vi "2023_day16_Task1.vi"() -> ()   [LabVIEW 2021]
uses:
  45de9bef-49e1-442e-b527-3241b48d18bf.vi
panel:
  out "Task 1":i32
  in  "Switch":bool caption="Ex. Data  vs.  User Data"
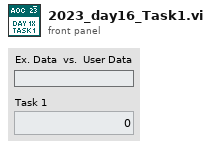
[diagram p1: front panel]
types:
  T1 = cluster{"Map":string[][], "Direction":enum16{"UP", "LEFT", "DOWN", "RIGHT"}, "Position (Row,Col)":i32[], "Energized Tiles":i32[][]}
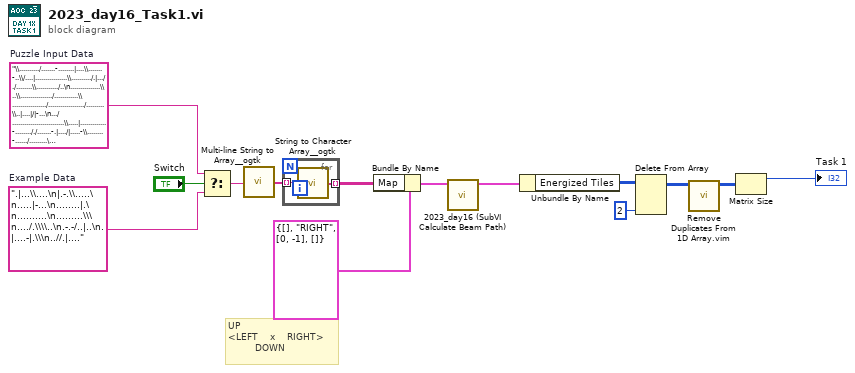
[diagram p0: block diagram]
diagram:
  w12 = "\\........../.......-........|....\\.......-..\\/....|................\\........../.|..././........\\.........../..\n...............\\..\\................/............\\................./................../.........\\..|....|/|-...\n.../..........................\\.....|.............-.......././.......-.|..../|.....-\\........-....../.........\n|..........................-..........-......./............................-..|................-..............\n.....|......../...../.......-.\\..............................-........|............|/.../../........./........\n..\\...|..-......\\.........-\\.||........|./................\\....\\........-..\\..................../..\\....-...|.\n.|...........|............-........./.-.................|.|....../...............|..../..-..-...\\...........|.\n..............\\............................................................./......................./\\....-...\n./........|...\\.\\..|..-....\\............................|........./.................|/...............-........\n\\....\\./.............../................../....|......./........../.\\......./........-....\\......../....../|..\n./......--..........\\..|.--........-...../......./........\\.....|/..................|//...........|.........-.\n.......|.....\\-.\\..-......-.........|.....................-/\\.....-..........|.............-....\\.....\\.-.....\n..--...\\....-..|..................................-......-......\\......-................\\...../..-/....--.....\n....-.........................\\.\\............|...............|.....-...\\....|-................................\n.................-..|.\\..\\....-..........|...../.....-...-.-../.............../................-..............\n-..-......|..............................\\.....\\........|...../........\\.................../..................\n..............-.....-.|..........|.\\..................|........|...........\\.\\...|........-...................\n..\\............/...\\\\........../...-..\\.../.........\\..|................../......\\..-.../....................\\\n..................|...\\......................./...|......../..............-./...\\........\\......./|...\\..-..-.\n.................................................-................|.........................................\\.\n......-...............................|./............./...........................-\\/..../......\\..........\\..\n......\\....|..........................\\.-|..........................|....................\\.....\\/...-.........\n..\\..-|...|.....-...../......./....|...............\\................|..|.......\\...........................-..\n..\\......-.......\\.........\\................|...........|....../...../..........-./...-|..................../.\n................./.......\\...|.....\\....-................./......../..\\...........-...|.../|................\\.\n..|..\\./.........\\.\\.......................-......|....-..../.../................-.......\\../.../...../.......\n........../........./..|..-....................\\\\............\\........................-......-......|.........\n.../-....\\..\\..........\\....\\\\......................................./........\\...-.................\\.........\n................................../.................|..\\.-..|................|/....-.........................|\n...-.................||..../....................-..........................................|.-................\n..//.\\..........................|.....|-.............\\.\\......-....\\.\\.......\\............-..............\\-...\n.......|.|..-........./..|........-.....|........................-...................-......\\................-\n..-..|..........|....-.............|.|/...../../..................\\...\\................../......|....|........\n........\\..././.............../.............../....-../.....|....\\................|/.../.....|.|-..|..........\n......|..........\\...-./........-...............................\\..........|.............|..\\..|......./.....|\n.............................-................................................|................/......\\.../..-\n......-........\\..........-..../...............\\............/.....\\......|........................-.|.../.....\n...\\...............-....-........-............-...../....|.\\.../.......\\..-....................|........|.....\n.............................-...\\....|...|.......\\............................-............\\.................\n....................|...-........-.........-..\\................/....................../.|.......-.............\n......\\.........................../....-....|...........................................\\...-.........|......\\\n.............\\../\\..............|\\.\\..........|\\.../..................../\\...................|\\.......\\.......\n/.................../.\\\\.........................../...........-...-..........-..-............................\n............\\......../........-.........../........./.................-................./...........|.........\n.........\\.......|.......\\........./.....................\\..............\\\\....../...|-....\\..|..-.....|.......\n.|....-.............\\.........\\.\\../.......-...........................\\./..........................--\\......\\\n........./..../................./.................\\............................................./../.\\........\n.....-..............-.-...\\/..|....-........./.....................\\................./.\\..........-...|....|..\n........|...|.-.......|.......-............\\.../....|...\\............../............-.........................\n........................|.....\\........................./\\/.........................|.........................\n....\\..././..........|.....\\......................-................./.....|...............................|-..\n.../.........../.-......\\..../.................-...\\.....-......\\.....\\..............//.|..............-..-...\n....../............./-/.\\...........\\...\\..|/........................-...../......\\........-./\\..........||...\n.................................../............|....................../..|.....\\......\\............/.........\n.....|....\\...|.-./............................./..-....|.\\.......................-../.-..-.........\\.........\n..........\\...|../.......-|............-........../...../..........-......-../.-......|..../.-.../............\n.-.........-............|/.......-........|...................-.........-........../.-........\\..........|/...\n.........\\.........\\....../....|...\\\\......-..........-................\\................................-.....\n............-...../......|...//........\\-....|......../........./..................-................../....--.\n...............|.................................|.../...\\....................\\................|...\\.|........\n..............\\.........\\.........\\....|.-.......\\.\\........-.........../...|.....|..............\\.......\\....\n........-.-.....|.../......-\\..|.....-.........|.-................\\......./....\\...-.....\\..|/...............|\n....|.....................-...................\\......\\......-.......................-...../........./....\\....\n..|...|.......\\./..-..............\\.............................................\\../....|.....................\n..................-../........|.....-\\.../................................................./..\\...|......-...-\n.....\\......\\........\\.....................|...|../......../....../.\\........./...............................\n............../........../...........\\..\\/..|.\\...|..........-................................\\-..............\n/...............\\...|......\\............/|...................|....././...\\............................-.|.....\n...........|................/-......\\.....-.........-.............../......./............../|.................\n..-...........|..\\.............\\....|/...............|..../..............\\...............|./......|........./.\n.....\\\\..|......\\....\\.......-.................\\.-......................|........./...|.........|...|...-.....\n-...../....|....../............./.......|/../\\.............../...../-\\.../-.......|........../..............\\\\\n..........\\....................../.................|...--../..................................................\n.\\.................../......|......-.............................//......|.../|.|....\\.............\\..........\n.\\-...........-.........|..................................../........|......../...-............\\....-...-....\n......\\......|................-...../....|........-..\\.....-........//................../.....|.........-.....\n.....-..........-.|/.........-....................../......|.|./........................................./\\\\|.\n...\\................|.........../..-....|..-..........|........../....-....../......./.....-..\\.....\\\\..../...\n.....\\.....-..................-...-..../....|....|.................|...\\./.............../.......|.\\/...../...\n.||......../........../.-...|...........\\.................\\........-........|........................-...|....\n........./......\\......|...............\\.\\.................................................\\.................|\n..........................|....................|..../-...............|....|......../....-..................|..\n.-........\\.|......../...|...................|.........|............\\.....|.......\\........./.................\n................-........................\\...........|................../................-.............\\......\n.......\\..........|.............../...|.-......................../....\\.............-.......\\./...............\n..........\\...........................................-........|.......\\........./...-........\\...............\n../......./...\\|...............-........\\................./...\\...................../.....-.-....-...........-\n.\\../......../....-\\................................|.....-..|...............................-................\n..........................\\.....|................/.....\\......../.............|..............\\......./-..|....\n|.........-.|............./......-.................|.......|...\\/...........|...........................\\\\....\n-..................|.........................-.............-.....|..../.........\\...-/.....|............/\\....\n.........\\.\\....\\...........|....-.../..............|.....|-.......\\.............-......./......././.......\\..\n..../.....-...........................................\\.../..\\.|.......................-..//....-......|......\n./-..................\\..\\....................................\\......./.\\....|.................................\n...../....................................-....-/........................-/.........-.\\...|......./..-.\\......\n.....|.............-.......|-..-.................................|-...........................\\.|.....|.......\n.........\\-.............\\.............../....-....|....-.|..........\\............|.\\...|.....-................\n............/.......-....|./....|../..../......./..\\.................-..................|.....................\n../....-........./.....\\...............\\......-....|...\\........../.....|........................\\............\n...../.\\.............\\.........................-..|.......|......-......|................./......./-..........\n...\\..........\\.......................\\.-..././.........|..\\..................\\...../...|.......|............-\n........./............-..................................|.....................-..............................\n........................|.....\\.........\\..............-..\\..........||...../.\\\\./....../.....................\n.................-.............\\.../...........\\...\\......--................\\.....\\.............\\....-........\n.../-..........\\.\\............-.......-.............\\..\\.\\...../........|...-..-..|..........\\................\n\\.|..\\......\\-......./.........||..\\.........................................................-...../..........\n....|..........................................\\......-..........\\.../...\\-........|..........................\n.......-.......\\..//./....|...............\\.\\..-...\\....|....................-......\\......\\..-......../......\n/..../../....-../....-....-......................\\........./..........-/..\\......./..\\-.../..........|........\n.|....\\\\........./....\\.............-......--\\...........|.........|..\\...................../........./.\\....."  # Puzzle Input Data
  w13 = ".|...\\....\n|.-.\\.....\n.....|-...\n........|.\n..........\n.........\\\n..../.\\\\..\n.-.-/..|..\n.|....-|.\\\n..//.|...."  # Example Data
  # "UP\n<LEFT    x    RIGHT>  \n         DOWN"
  n1 = Select(t=w12, s="Switch", f=w13) -> (s? t:f=w11:string)
  n2 = call <userlib>:"Multi-line String to Array__ogtk.vi"("string"=w11) -> ("lines"=w10:string[])
  n3 = for {
    tunnel: w10 -> [w16] mode=indexing
    tunnel: [w15] -> w6 mode=indexing
    n4 = call <userlib>:"String to Character Array__ogtk.vi"("Input String"=w16) -> ("Character Array"=w15:string[])
  }
  n5 = Bundle By Name(cluster=T1 {"Map"=[], "Direction"=enum."RIGHT", "Position (Row,Col)"=[0, -1], "Energized Tiles"=[]} ("Beam"), "Map"=w6) -> (w8:T1)
  n6 = call "2023_day16 (SubVI Calculate Beam Path).vi"("Beam in"=w8) -> ("Beam out"=w7:T1)  [unwired: 10 in]
  n7 = Unbundle By Name(w7) -> ("Energized Tiles"=w1:i32[][])
  n8 = Delete From Array(array=w1, index (col)=2 ("disabled index (col)")) -> (array with subset deleted=w3:i32[][])  [unwired: 2 in, 1 out]
  n9 = call "Remove Duplicates From 1D Array.vim"("array"=w3) -> ("array with duplicates removed"=w5:i32[][])  [unwired: 10 in]
  n10 = Matrix Size(0:w5) -> (1:→"Task 1":i32)  [unwired: 1 out]
